vi "WPI_SimpleGyroLoop.vi"(8 "error in":errorcluster, 11 "SimpleGyroDevRef":T1) -> ()   [LabVIEW 2014, in "SimpleGyro.lvlib"]
uses:
  SimpleGyro.lvlib
  WPI_SimpleGyroDevRef.ctl
  <vilib>/Rock Robotics/SystemInterfaces/Typedef/FPGA_TypedefDigitalModule.ctl
  <vilib>/Rock Robotics/SystemInterfaces/spilib/spi_bus.ctl
  <vilib>/Rock Robotics/WPI/SPI/WPI_SPIDevRef.ctl
  <vilib>/Platform/TimedLoop/XDataNode/timing_clust.ctl
  <vilib>/Platform/TimedLoop/XDataNode/nitl_modes.ctl
  <vilib>/Platform/TimedLoop/XDataNode/wakeup.ctl
  <vilib>/platform/TimedLoop/XDataNode/XDataNode.xnode
  <vilib>/Platform/TimedLoop/XDataNode/XDNodeRunTimeDep.lvlib
  <vilib>/ptbypt/NI_PtbyPt.lvlib
panel:
  out "mean":dbl format="%0.2f"
  in  "Calibrate":bool
  out "Angle":dbl
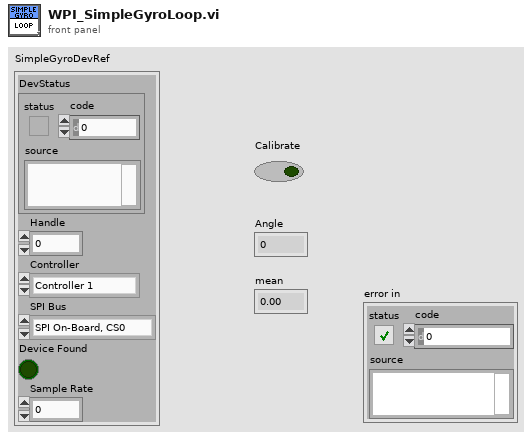
[diagram p1: front panel]
types:
  T1 = typedef "SimpleGyro.lvlib/WPI_SimpleGyroDevRef.ctl" = cluster{"DevStatus":errorcluster, "Handle":i32, "Controller":T2, "SPI Bus":T3, "Device Found":bool, "Sample Rate":dbl}
  T2 = typedef "FPGA_TypedefDigitalModule.ctl" = enum16{"Controller 1"}
  T3 = typedef "spi_bus.ctl" = enum16{"SPI On-Board, CS0", "SPI On-Board, CS1", "SPI On-Board, CS2", "SPI On-Board, CS3", "SPI MXP", "Invalid"}
  T4 = typedef "WPI_SPIDevRef.ctl" = cluster{"DevStatus":errorcluster, "Handle":i32, "Controller":T2, "SPI Bus":T3}
  T5 = typedef "XDNodeRunTimeDep.lvlib/timing_clust.ctl" = cluster{"Expected End [f-1]":u64, "Actual End [f-1]":u64, "Finished Late? [f-1]":bool, "Expected End [i-1]":u64, "Actual End [i-1]":u64, "Finished Late? [i-1]":bool, "Expected Start [i]":u64, "Actual Start [i]":u64, "Expected Start [f]":u64, "Actual Start [f]":u64, "Source Name":string, "Structure Name":string, "Period":i64, "Deadline":i64, "Offset":i64, "Start":i64, "Priority":i32, "Timeout":i32, "Mode":T6, "Wakeup Reason":T7, "Error":errorcluster, "Source Type":string, "Secondary Source Type":string, "Global End Time":u64, "Global Start Time":u64, "Frame Duration":u64, "Iteration Duration":u64, "Assigned CPU":i32, "I/O Scan Engine Mode":u32}
  T6 = typedef "XDNodeRunTimeDep.lvlib/nitl_modes.ctl" = enum32{"No Change", "Process missed periods, maintain original phase", "Discard missed periods, maintain original phase", "Process missed periods, ignore original phase", "Discard missed periods, ignore original phase"}
  T7 = typedef "XDNodeRunTimeDep.lvlib/wakeup.ctl" = enum32{"Normal", "Aborted", "Asynchronous wakeup", "Timing source error", "Timed loop error", "Timeout"}
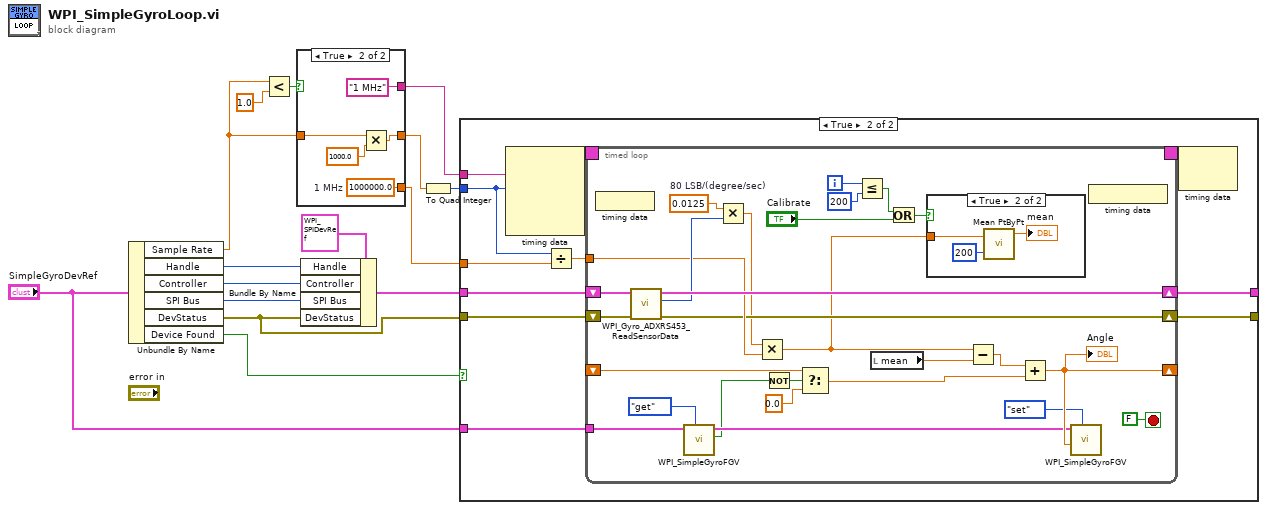
[diagram p0: block diagram]
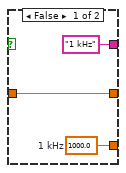
[diagram p2: hidden frame]
diagram:
  n1 = Unbundle By Name("SimpleGyroDevRef") -> ("Sample Rate"=w5:dbl, "Handle"=w14:i32, "Controller"=w13:T2, "SPI Bus"=w12:T3, "DevStatus"=w10:errorcluster, "Device Found"=w9:bool)
  n2 = Less?(x=w5, y=1.0) -> (x < y?=w7:bool)
  n3 = case shown="True" w7 {
    tunnel: ["1 kHz" ("Source Name") "1 MHz" ("Source Name")] -> w6
    tunnel: w5 -> [w18 w22]
    tunnel: [w18 w21] -> w4
    tunnel: [w16 w19] -> w2
    frame False {
      w16 = 1000.0  # 1 kHz
    }
    frame True {
      w19 = 1000000.0  # 1 MHz
      n4 = Multiply(x=w22, y=1000.0) -> (x*y=w21:dbl)
    }
  }
  n5 = Bundle By Name(cluster=T4 {"DevStatus"={"status"=FALSE, "code"=0, "source"=""}, "Handle"=0, "Controller"=enum."Controller 1", "SPI Bus"=enum."Invalid"} ("SPIDevRef out"), "Handle"=w14, "Controller"=w13, "SPI Bus"=w12, "DevStatus"=w10) -> (w11:T4)
  n6 = To Quad Integer(1:w4) -> (0:w3:i64)
  n7 = case shown="True" w9 {
    tunnel: w11 -> [w25 w34]
    tunnel: w10 -> [w24 w33]
    tunnel: [w24 w32] -> _
    tunnel: [w25 w31] -> _
    tunnel: w6 -> [_ w29]
    tunnel: w3 -> [_ w28]
    tunnel: w2 -> [_ w27]
    tunnel: "SimpleGyroDevRef" -> [_ w26]
    frame False {
    }
    frame True {
      n8 = node-c288(w29, w28) -> (w36:T5)  [unwired: 2 in]
      n9 = Divide(x=w28, y=w27) -> (x/y=w30:dbl)
      n10 = timed-loop {
        shift-right: [w61] -> w31
        shift-left: w34 -> [w63]
        shift-right: [w56] -> w32
        shift-left: w33 -> [w62]
        timing: w36 -> [_]
        timing-out: [_] -> w35
        shift-right: [w40] -> _
        shift-left: _ -> [w58]
        tunnel: w30 -> [w57]
        tunnel: w26 -> [w42]
        i -> [w46]
        stop <- FALSE stop-if-true
        w59 = 0.0125  # 80 LSB/(degree/sec)
        n11 = node-c288() -> ()  [unwired: 1 in]
        n12 = call <vilib>:"WPI_Gyro_ADXRS453_ReadSensorData.vi"("error in (no error)"=w62, "SPIDevRef in"=w63) -> ("error out"=w56:errorcluster, "Sensor Data (n-1)"=w60:i16, "SPIDevRef out"=w61:T4)  [unwired: 5 in, 2 out]
        n13 = call "WPI_SimpleGyroFGV.vi"("Operation"=enum16{"set", "get"}."get", "SimpleGyroDevRef"=w42) -> ("Reset?"=w37:bool, "SimpleGyroDevRef"=w38:T1)  [unwired: 7 in, 1 out]
        n14 = Multiply(x=w59, y=w60) -> (x*y=w53:dbl)
        n15 = Multiply(x=w53, y=w57) -> (x*y=w52:dbl)
        n16 = Not(x=w37) -> (.not. x?=w43:bool)
        n17 = Select(t=w58, s=w43, f=0.0 ("t")) -> (s? t:f=w50:dbl)
        n18 = Less Or Equal?(x=w46, y=200) -> (x <= y?=w44:bool)
        n19 = local read "mean"() -> (w48:dbl)
        n20 = Or(x=w44, y="Calibrate") -> (x .or. y?=w47:bool)
        n21 = case shown="True" w47 {
          tunnel: w52 -> [_ w65]
          frame False {
          }
          frame True {
            n22 = call <vilib>:"Mean PtByPt.vi"("x"=w65, "sample length"=200) -> ("mean"=→"mean":dbl)  [unwired: 2 in, 1 out]
          }
        }
        n23 = Subtract(x=w52, y=w48) -> (x-y=w55:dbl)
        n24 = Add(x=w55, y=w50) -> (x+y=w40:dbl)
        "Angle" <- w40
        n25 = call "WPI_SimpleGyroFGV.vi"("Operation"=enum16{"set", "get"}."set", "Angle"=w40, "SimpleGyroDevRef"=w38) -> ()  [unwired: 6 in, 3 out]
        n26 = node-c288() -> ()  [unwired: 1 out]
      }
      n27 = node-c288(w35) -> ()  [unwired: 1 out]
    }
  }
